vi "Set String Value.vi"(8 "error in (no error)":errorcluster caption="错误输入（无错误）", 9 "Active Row Number":i32 caption="活动行数", 10 "Editing Path Ref":refnum<vi> caption="编辑路径引用", 11 "Include Paths Ref":refnum<vi> caption="包括路径引用") -> (0 "error out":errorcluster caption="错误输出", 2 "Dup Editing Path Ref":refnum<vi> caption="编辑路径引用副本", 3 "Dup Include Paths Ref":refnum<vi> caption="包括路径引用副本")   [LabVIEW 2011, in "NISAST Include Paths.xctl"]
uses:
  NISAST Include Paths.xctl
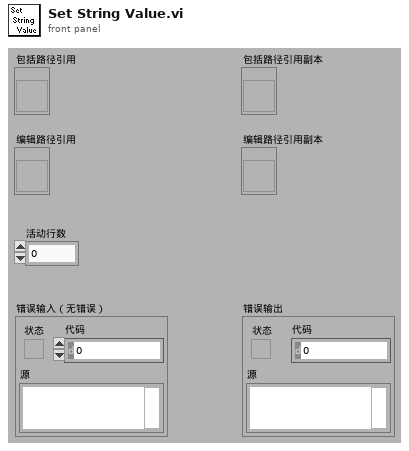
[diagram p1: front panel]
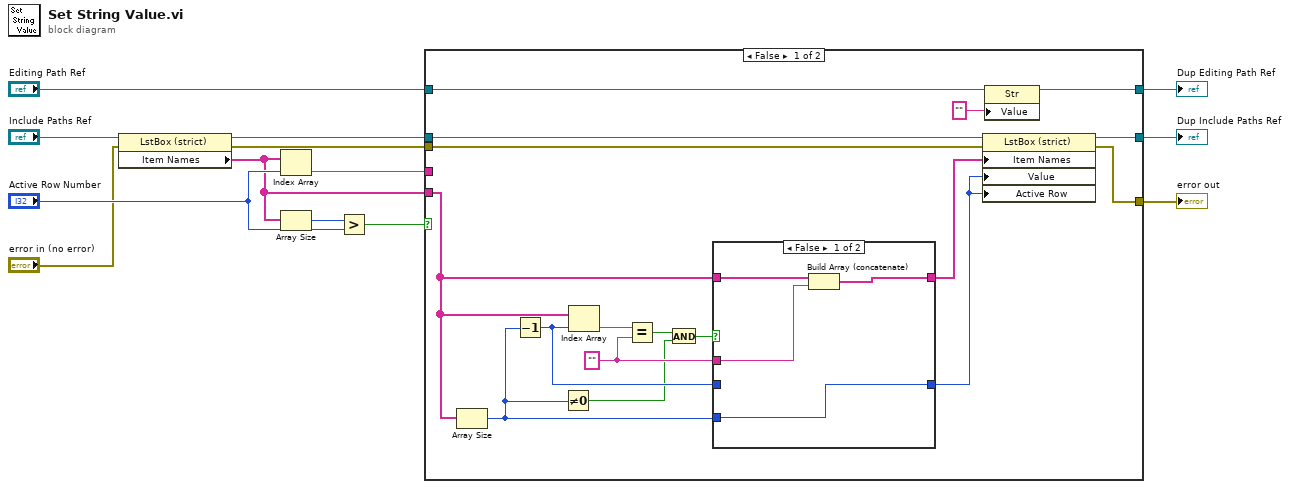
[diagram p0: block diagram]
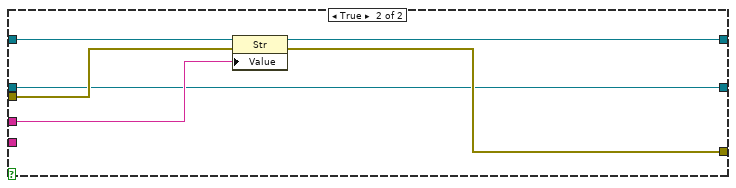
[diagram p3: hidden frame]
diagram:
  n1 = property class="LstBox (strict)"(reference="Include Paths Ref", error in="error in (no error)") -> (reference out=w5:refnum<vi>, error out=w7:errorcluster, "Item Names"=w2:string[])
  n2 = Index Array(array=w2, index="Active Row Number") -> (element=w11:string)
  n3 = Array Size(array=w2) -> (size(s)=w1:i32)
  n4 = Greater?(x=w1, y="Active Row Number") -> (0:w12:bool)
  n5 = case shown="False" w12 {
    tunnel: "Editing Path Ref" -> [w28 w42]
    tunnel: w11 -> [_ w41]
    tunnel: w7 -> [w24 w40]
    tunnel: [w25 w39] -> w6
    tunnel: w5 -> [w30 w37]
    tunnel: [w29 w37] -> w4
    tunnel: [w27 w38] -> w3
    tunnel: w2 -> [w21 _]
    frame False {
      w18 = ""
      n6 = Array Size(array=w21) -> (size(s)=w17:i32)
      n7 = Decrement(x=w17) -> (x-1=w23:i32)
      n8 = Not Equal To 0?(x=w17) -> (x != 0?=w14:bool)
      n9 = Index Array(array=w21, index=w23) -> (element=w22:string)
      n10 = Equal?(x=w22, y=w18) -> (x = y?=w16:bool)
      n11 = And(x=w16, y=w14) -> (x .and. y?=w15:bool)
      n12 = case shown="False" w15 {
        tunnel: [w34 w35] -> w20
        tunnel: w21 -> [w33 w35]
        tunnel: [w32 w36] -> w19
        tunnel: w17 -> [w32 _]
        tunnel: w23 -> [_ w36]
        tunnel: w18 -> [w31 _]
        frame False {
          n13 = Build Array (concatenate)(w33, w31) -> (w34:string[])
        }
        frame True {
        }
      }
      n14 = property class="LstBox (strict)"(reference=w30, error in=w24, "Item Names"=w20, "Value"=w19, "Active Row"=w19) -> (reference out=w29:refnum<vi>, error out=w25:errorcluster)
      n15 = property class="Str"(reference=w28, "Value"="") -> (reference out=w27:refnum<vi>)  [unwired: 1 in, 1 out]
    }
    frame True {
      n16 = property class="Str"(reference=w42, error in=w40, "Value"=w41) -> (reference out=w38:refnum<vi>, error out=w39:errorcluster)
    }
  }
  "Dup Editing Path Ref" <- w3
  "error out" <- w6
  "Dup Include Paths Ref" <- w4
